vi "Drive Immediate.vi"(7 "Description":string, 8 "Command Info In":T1, 9 "Right joystick x":dbl, 10 "Left joystick y":dbl, 11 "Left joystick x":dbl) -> (0 "Command Info Out":T1)   [LabVIEW 2019]
doc: "Often used for joystick control, this VI checks to see that the joystick axes are outside the deadband and updates the motors appropriately."
uses:
  <vilib>/Rock Robotics/WPI/Framework/Command Status Info.ctl
  <vilib>/Rock Robotics/WPI/Framework/Completion Status.ctl
  <vilib>/Rock Robotics/WPI/Framework/Completion Notifier.ctl
  Implementation/Drive Setpoints.ctl
  Implementation/Drive Operations.ctl
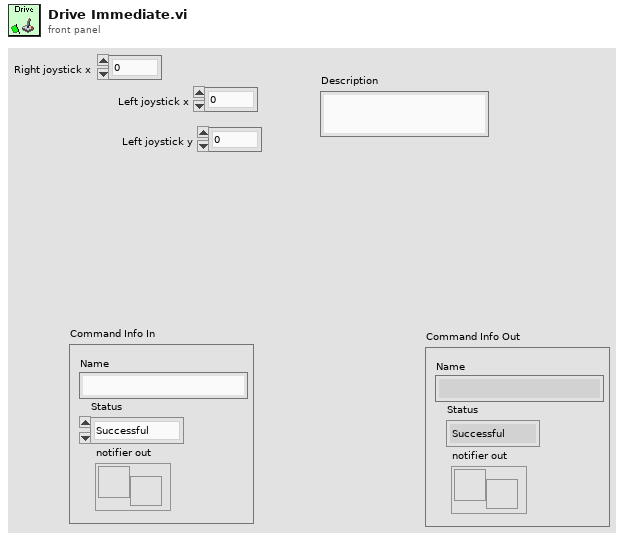
[diagram p1: front panel]
types:
  T1 = typedef "Command Status Info.ctl" = cluster{"Name":string, "Status":T2, "notifier out":T3}
  T2 = typedef "Completion Status.ctl" = enum16{"Successful", "Aborted", "Incomplete"}
  T3 = typedef "Completion Notifier.ctl" = refnum<notifier>
  T4 = typedef "Drive Setpoints.ctl" = cluster{"Operation":T5, "Left joystick x":dbl, " Right joystick x":dbl, "Left joystick y":dbl}
  T5 = typedef "Drive Operations.ctl" = enum16{"Reserve", "Sniper Drive", "Set Initial Heading", "Read Current", "Immediate", "Drive for Time", "Drive for Distance"}
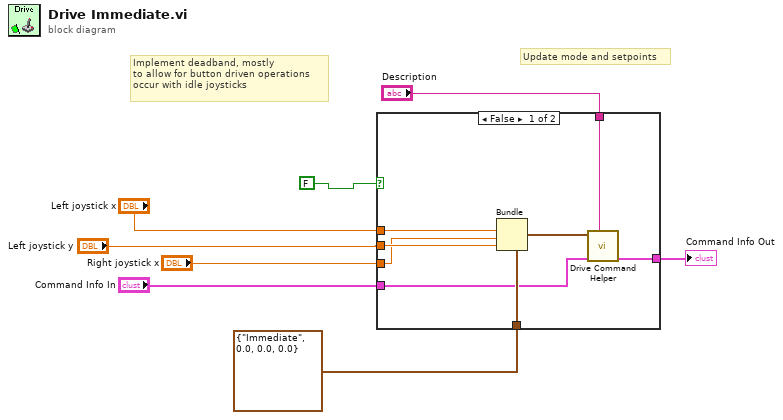
[diagram p0: block diagram]
diagram:
  # "Implement deadband, mostly\nto allow for button driven operations\noccur with idle joysticks"
  # "Update mode and setpoints"
  n1 = case shown="False" FALSE {
    tunnel: "Left joystick x" -> [w16 _]
    tunnel: T4 {"Operation"=enum."Immediate", "Left joystick x"=0.0, " Right joystick x"=0.0, "Left joystick y"=0.0} ("SubSystem Data") -> [w15 _]
    tunnel: [w14 w17] -> w8
    tunnel: "Command Info In" -> [w13 w17]
    tunnel: "Description" -> [w11 _]
    tunnel: "Left joystick y" -> [w10 _]
    tunnel: "Right joystick x" -> [w9 _]
    frame False {
      n2 = Bundle(cluster=w15, "Left joystick x"=w16, "Right joystick x"=w9, "Left joystick y"=w10) -> (w12:T4)  [unwired: 1 in]
      n3 = call "Drive Command Helper.vi"("Description"=w11, "Command Info In"=w13, "SubSystem Data"=w12) -> ("Command Info Out"=w14:T1)  [unwired: 6 in, 2 out]
    }
    frame True {
    }
  }
  "Command Info Out" <- w8
